vi "AMX-SaveImage.vi"(0 "基路径":path, 1 "CCD Name":string(combo), 5 "布尔":bool=TRUE, 7 "结果":bool=TRUE, 9 "Image in":T1(plugin-control), 11 "error in (no error)":errorcluster, 13 "类型":string(combo)="Front conveyor") -> (15 "error out":errorcluster)   [LabVIEW 2017]
panel:
  out "连接的字符串":string
  # "D:\\Data\\History Image\\20190228\\CCD3\\Image"
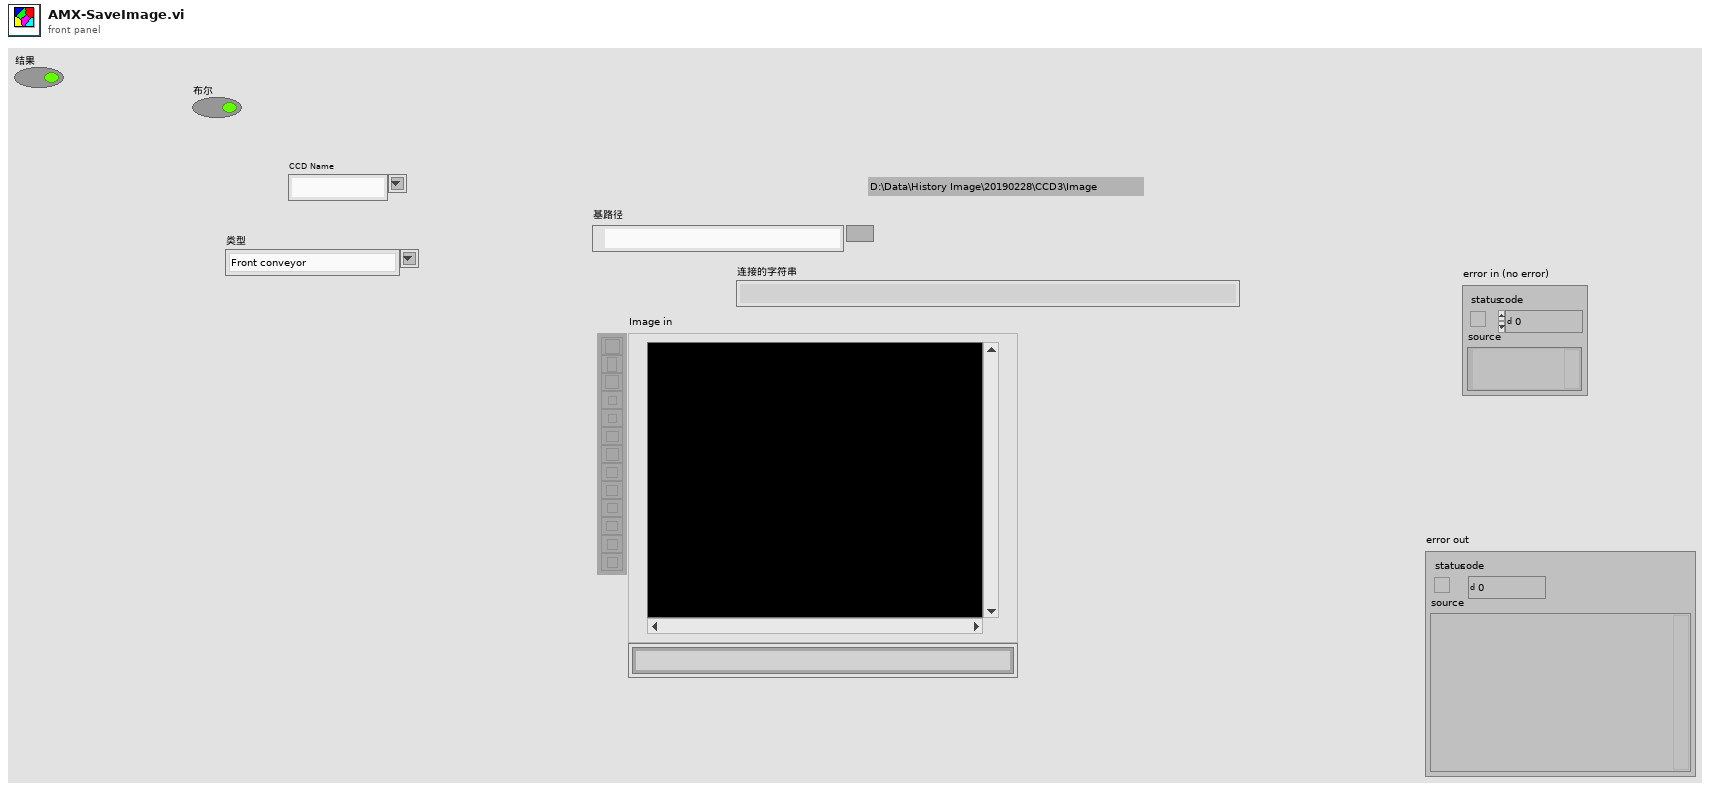
[diagram p1: front panel]
types:
  T1 = typedef "IMAQ Image.ctl" = refnum<image>
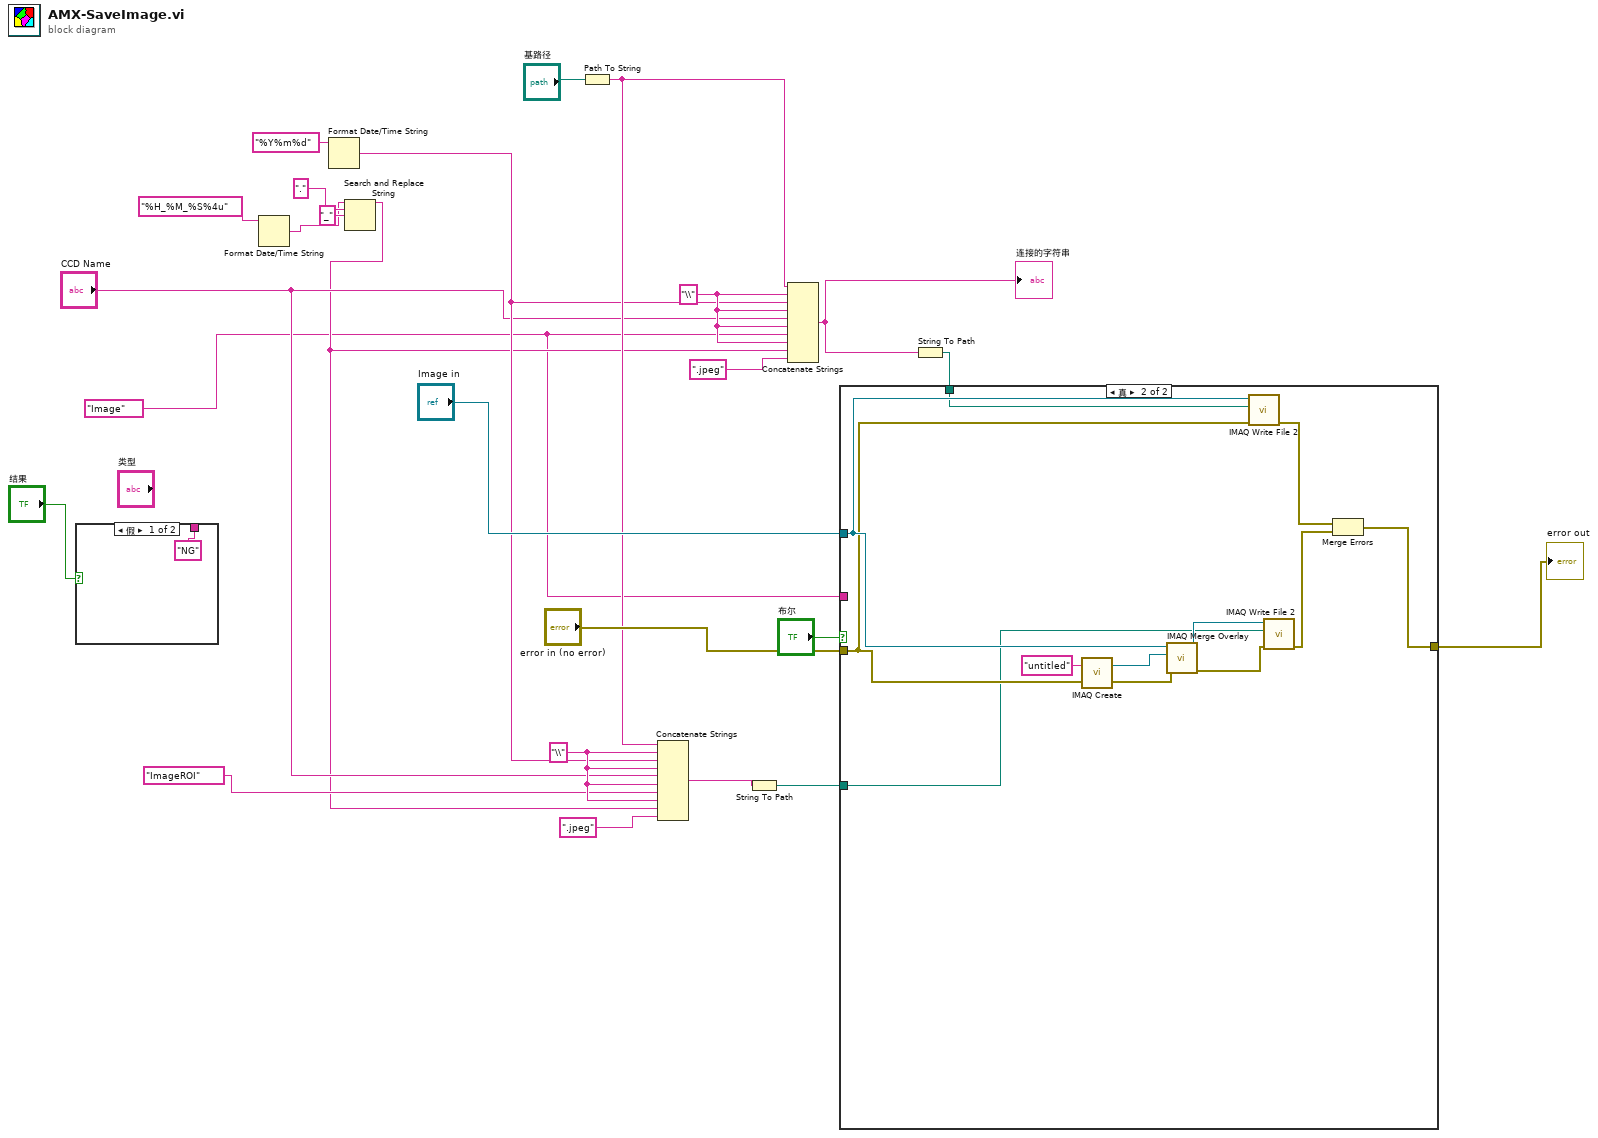
[diagram p0: block diagram]
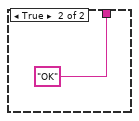
[diagram p2: hidden frame]
diagram:
  w2 = "Image" ("类型")
  w15 = "\\" ("字符串")
  w17 = "\\" ("字符串")
  n1 = case shown="假" "结果" {
    tunnel: ["NG" "OK"] -> _
    frame False {
    }
    frame True {
    }
  }
  n2 = Format Date/Time String(time format string (%c)="%H_%M_%S%4u" ("时间格式字符串(%c)")) -> (date/time string=w5:string)  [unwired: 2 in]
  n3 = Format Date/Time String(time format string (%c)="%Y%m%d" ("时间格式字符串(%c)")) -> (date/time string=w12:string)  [unwired: 2 in]
  n4 = Search and Replace String(input string=w5, search string="." ("搜索字符串"), replace string="_" ("替换字符串(\"\")")) -> (result string=w4:string)  [unwired: 5 in, 3 out]
  n5 = Path To String(path="基路径") -> (string=w13:string)
  n6 = Concatenate Strings(w13, w15, w12, w15, "CCD Name", w15, "ImageROI" ("类型"), w15, w4, ".jpeg" ("字符串")) -> (w9:string)
  n7 = String To Path(string=w9) -> (path=w8:path)
  n8 = Concatenate Strings(w13, w17, w12, w17, "CCD Name", w17, w2, w17, w4, ".jpeg" ("字符串")) -> (w23:string)
  "连接的字符串" <- w23
  n9 = String To Path(string=w23) -> (path=w19:path)
  n10 = case shown="真" "布尔" {
    tunnel: "Image in" -> [_ w40]
    tunnel: "error in (no error)" -> [w28 w39]
    tunnel: w19 -> [_ w29]
    tunnel: [w28 w31] -> w1
    tunnel: w2 -> [_ _]
    tunnel: w8 -> [_ w30]
    frame False {
    }
    frame True {
      n11 = call "IMAQ Create"("Image Name"="untitled", "error in (no error)"=w39) -> ("New Image"=w35:T1, "error out"=w34:errorcluster)  [unwired: 3 in]
      n12 = call "IMAQ Merge Overlay"("error in (no error)"=w34, "Image Dst"=w35, "Image Src"=w40) -> ("error out"=w37:errorcluster, "Image Dst Out"=w38:T1)  [unwired: 7 in]
      n13 = call-poly "IMAQ Write File 2"("error in (no error)"=w39, "File Path"=w29, "Image"=w40) -> ("error out"=w32:errorcluster)  [unwired: 7 in, 1 out]
      n14 = call-poly "IMAQ Write File 2"("error in (no error)"=w37, "File Path"=w30, "Image"=w38) -> ("error out"=w33:errorcluster)  [unwired: 7 in, 1 out]
      n15 = Merge Errors(w32, w33) -> (w31:errorcluster)
    }
  }
  "error out" <- w1
